vi "Loop Check.vi"(0 "Pause":bool, 1 "Stop":bool) -> (2 "Pause":bool, 3 "State":string, 4 "ABORT":bool)   [LabVIEW 2020]
doc: "Checks the pause and stop buttons in a loop.\nScott Hannahs, FBNML, Jan 1992"
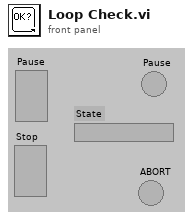
[diagram p1: front panel]
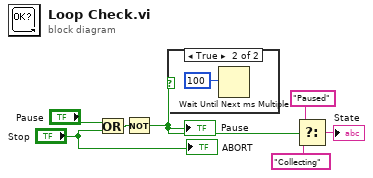
[diagram p0: block diagram]
diagram:
  n1 = Or(x="Pause", y="Stop") -> (x .or. y?=w7:bool)
  n2 = Not(x=w7) -> (.not. x?=w4:bool)
  "Pause" <- w4
  n3 = case shown="True" w4 {
    frame False {
    }
    frame True {
      n4 = Wait Until Next ms Multiple(millisecond multiple=u32 100) -> ()  [unwired: 1 out]
    }
  }
  n5 = Select(t="Paused", s=w4, f="Collecting") -> (s? t:f=→"State":string)
  "ABORT" <- "Stop"
